vi "Untitled 1.vi"() -> ()   [LabVIEW 2019]
uses:
  <vilib>/sound2/lvsound2.llb/Sound Data Format.ctl
  <vilib>/sound2/lvsound2.llb/Sampling Mode.ctl
  <vilib>/Analysis/2dsp.llb/Real FFT.vi
  <vilib>/sound2/lvsound2.llb/Sound Input Read (DBL).vi
  <vilib>/Analysis/NI_AALPro.lvlib
  func.dll
panel:
  in  "Threshold":dbl
  out "Array":dbl[](array[numeric])
  out "range":i32
  out "duration":i32
  out "f1":i32
  out "f0":i32
  out "array_length":i32
  out "type":i32
  out "array_pow":i32[](array[numeric])
  out "array_indice 2":i32[](array[numeric])
  out "Waveform Graph 2":dbl[](graph)
  out "Waveform Graph":waveform(dbl)[](graph)
  in  "sound format":T1={"sample rate (S/s)"=22050.0, "number of channels"=2, "bits per sample"=16}
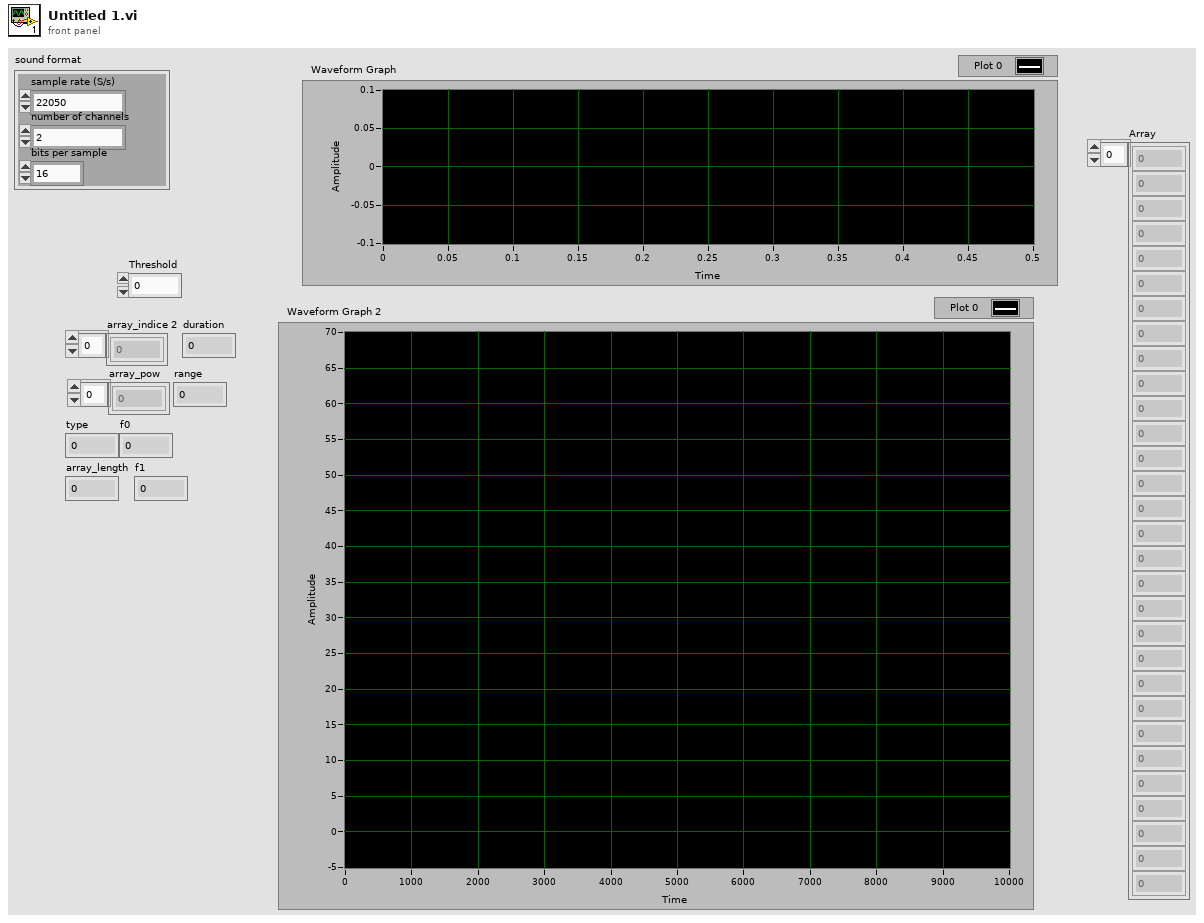
[diagram p1: front panel]
types:
  T1 = typedef "Sound Data Format.ctl" = cluster{"sample rate (S/s)":dbl, "number of channels":i32, "bits per sample":i32}
  T2 = typedef "Sampling Mode.ctl" = i32
  T3 = typedef "Sound Input Task ID.ctl" = u32
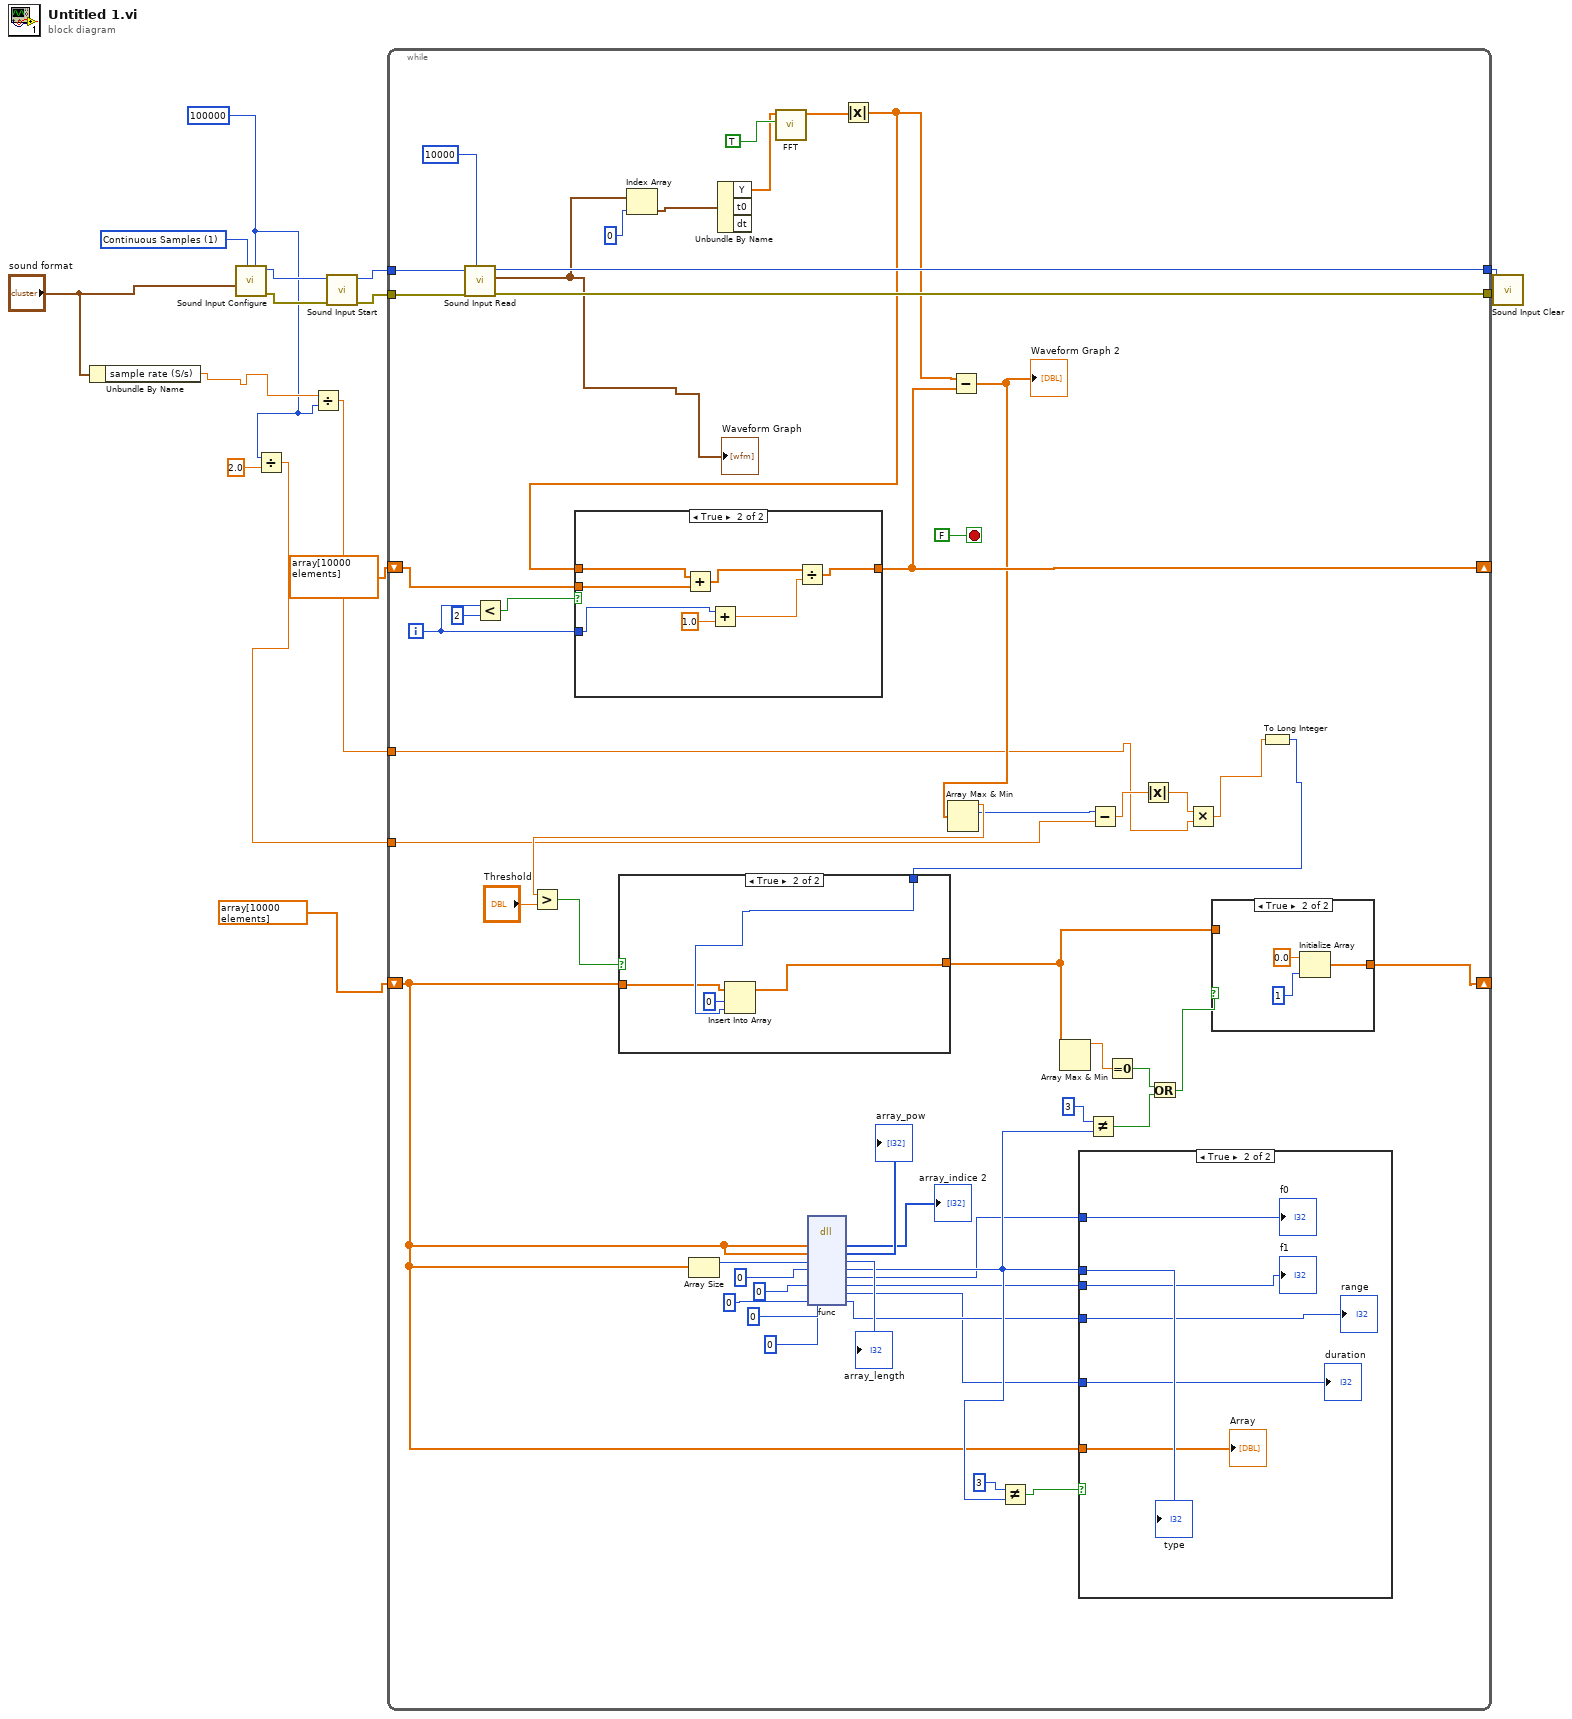
[diagram p0: block diagram]
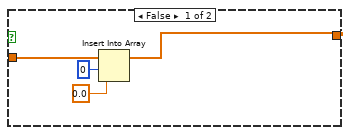
[diagram p4: hidden frame]
diagram:
  w15 = T2 1 items=["Finite Samples", "Continuous Samples"] ("sample mode")
  w3 = 100000 ("number of samples/ch")
  n1 = Unbundle By Name("sound format") -> ("sample rate (S/s)"=w5:dbl)
  n2 = call <vilib>:"Sound Input Configure.vi"("number of samples/ch"=w3, "sample mode"=w15, "sound format"="sound format") -> ("error out"=w14:errorcluster, "task ID"=w13:T3)  [unwired: 7 in]
  n3 = Divide(x=w3, y=2.0) -> (x/y=w2:dbl)
  n4 = Divide(x=w5, y=w3) -> (x/y=w1:dbl)
  n5 = call <vilib>:"Sound Input Start.vi"("error in (no error)"=w14, "task ID"=w13) -> ("error out"=w11:errorcluster, "task ID out"=w12:T3)  [unwired: 8 in]
  n6 = while {
    tunnel: w12 -> [w68]
    tunnel: w11 -> [w67]
    tunnel: [w65] -> w10
    tunnel: [w64] -> w9
    shift-right: [w51] -> _
    shift-left: dbl[] array[10000 elements] -> [w56]
    shift-right: [w37] -> _
    shift-left: dbl[] array[10000 elements] -> [w23]
    tunnel: w2 -> [w21]
    tunnel: w1 -> [w18]
    i -> [w55]
    stop <- FALSE stop-if-true
    n7 = call-poly <vilib>:"Sound Input Read.vi"("number of samples/ch"=10000, "error in (no error)"=w67, "task ID"=w68) -> ("error out"=w64:errorcluster, "data"=w62:waveform(dbl)[], "task ID out"=w65:T3)  [unwired: 6 in]
    "Waveform Graph" <- w62
    n8 = Less?(x=w55, y=2) -> (x < y?=w53:bool)
    n9 = Index Array(array=w62, index=0) -> (element=w60:waveform(dbl))
    n10 = Array Size(array=w23) -> (size(s)=w44:i32)
    n11 = Unbundle By Name(w60) -> ("Y"=w57:dbl[])  [unwired: 2 out]
    n12 = call-poly <vilib>:"FFT.vi"("shift?"=TRUE, "X"=w57) -> ("FFT {X}"=w58:cdb[])  [unwired: 8 in, 1 out]
    n13 = dll-call lib="C:/Users/bilge/Documents/proje/func.dll" fn="func"("array_indice"=w23, "array_pow"=w23, "array_length"=w44, "type"=0, "f0"=0, "f1"=0, "duration"=0, "range"=0) -> ("array_indice"=→"array_indice 2":i32[], "array_pow"=→"array_pow":i32[], "array_length"=→"array_length":i32, "type"=w29:i32, "f0"=w27:i32, "f1"=w26:i32, "duration"=w25:i32, "range"=w28:i32)  [unwired: 4 in, 2 out]
    n14 = Absolute Value(x=w58) -> (abs(x)=w52:dbl[])
    n15 = case shown="True" w53 {
      tunnel: w52 -> [_ w94]
      tunnel: [w87 w88] -> w51
      tunnel: w56 -> [w87 w93]
      tunnel: w55 -> [_ w91]
      frame False {
      }
      frame True {
        n16 = Add(x=w94, y=w93) -> (x+y=w89:dbl[])
        n17 = Add(x=w91, y=1.0) -> (x+y=w90:dbl)
        n18 = Divide(x=w89, y=w90) -> (x/y=w88:dbl[])
      }
    }
    n19 = Subtract(x=w52, y=w51) -> (x-y=w50:dbl[])
    "Waveform Graph 2" <- w50
    n20 = Array Max & Min(array=w50) -> (max value=w49:dbl, max index (indices)=w22:i32)  [unwired: 2 out]
    n21 = Greater?(x=w49, y="Threshold") -> (0:w48:bool)
    n22 = Not Equal?(x=3, y=w29) -> (x != y?=w30:bool)
    n23 = case shown="True" w30 {
      tunnel: w29 -> [_ w74]
      tunnel: w28 -> [_ w73]
      tunnel: w27 -> [_ w72]
      tunnel: w26 -> [_ w71]
      tunnel: w25 -> [_ w70]
      tunnel: w23 -> [_ w69]
      frame False {
      }
      frame True {
        "type" <- w74
        "range" <- w73
        "f0" <- w72
        "f1" <- w71
        "duration" <- w70
        "Array" <- w69
      }
    }
    n24 = Not Equal?(x=3, y=w29) -> (x != y?=w33:bool)
    n25 = Subtract(x=w22, y=w21) -> (x-y=w20:dbl)
    n26 = Absolute Value(x=w20) -> (abs(x)=w19:dbl)
    n27 = Multiply(x=w19, y=w18) -> (x*y=w17:dbl)
    n28 = To Long Integer(number=w17) -> (32bit integer=w16:i32)
    n29 = case shown="True" w48 {
      tunnel: [w81 w85] -> w36
      tunnel: w16 -> [_ w84]
      tunnel: w23 -> [w80 w83]
      frame False {
        n30 = Insert Into Array(array=w80, index=0, new element=0.0 ("new element/subarray")) -> (w81:dbl[])
      }
      frame True {
        n31 = Insert Into Array(array=w83, index=0, new element=w84) -> (w85:dbl[])
      }
    }
    n32 = Array Max & Min(array=w36) -> (max value=w38:dbl)  [unwired: 3 out]
    n33 = Equal To 0?(x=w38) -> (x = 0?=w34:bool)
    n34 = Or(x=w34, y=w33) -> (x .or. y?=w32:bool)
    n35 = case shown="True" w32 {
      tunnel: [w75 w76] -> w37
      tunnel: w36 -> [w75 _]
      frame False {
      }
      frame True {
        n36 = Initialize Array(0.0 ("element"), 1 ("dimension size")) -> (w76:dbl[])
      }
    }
  }
  n37 = call <vilib>:"Sound Input Clear.vi"("error in (no error)"=w9, "task ID"=w10) -> ()  [unwired: 9 in, 1 out]
